vi "Instantiate.vi"(8 "error in":errorcluster, 10 "gRPCid":T1, 11 "iService":refnum<class "ServiceBase.lvclass">) -> (0 "error out":errorcluster, 3 "iService":refnum<class "ServiceBase.lvclass">)   [LabVIEW 2019, in "gRPC-servicer.lvlib" / "ServiceBase.lvclass"]
uses:
  ServiceBase.lvclass
  <vilib>/gRPC/LabVIEW gRPC Library/Shared/grpcId.ctl
  <vilib>/gRPC/LabVIEW gRPC Library/grpc-lvsupport-release.lvlib
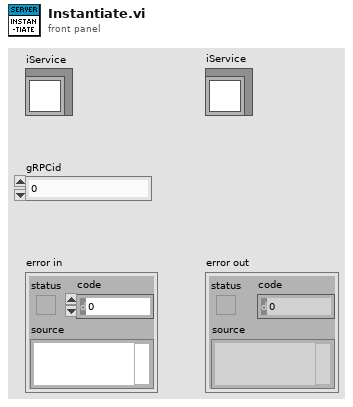
[diagram p1: front panel]
types:
  T1 = typedef "grpc-lvsupport-release.lvlib/grpcId.ctl" = u64
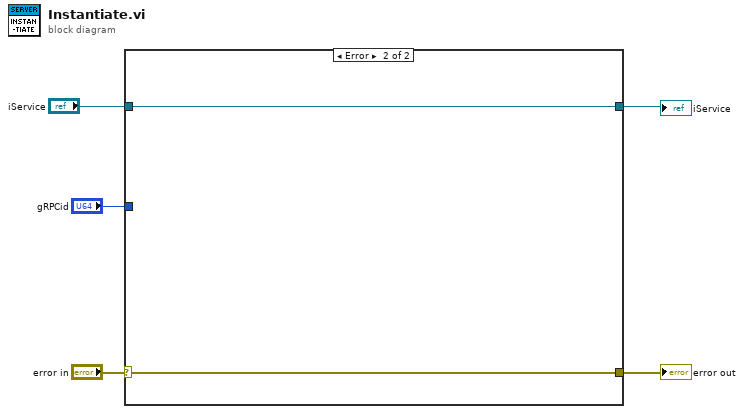
[diagram p0: block diagram]
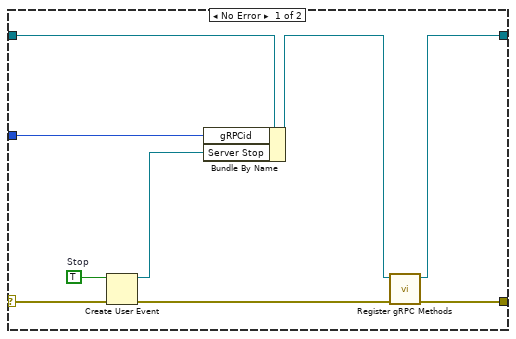
[diagram p2: hidden frame]
diagram:
  n1 = case shown="Error" "error in" {
    selector: "error in" -> [w14 w16]
    tunnel: [w12 w16] -> w4
    tunnel: [w7 w15] -> w3
    tunnel: "gRPCid" -> [w6 _]
    tunnel: "iService" -> [w9 w15]
    frame No Error {
      w11 = TRUE  # Stop
      n2 = Create User Event(user event datatype=w11, error in=w14) -> (user event=w10:refnum<user-event>, error out=w13:errorcluster)
      n3 = Bundle By Name(cluster=w9, "gRPCid"=w6, "Server Stop"=w10) -> (w8:refnum<class "ServiceBase.lvclass">)
      n4 = call-dynamic "Register gRPC Methods.vi"("error in"=w13, "Template Server in"=w8) -> ("error out"=w12:errorcluster, "Template Server out"=w7:refnum<class "ServiceBase.lvclass">)  [unwired: 8 in]
    }
    frame Error {
    }
  }
  "error out" <- w4
  "iService" <- w3
